vi "ResetDirection.vi"(8 "error in":errorcluster, 11 "class data in":refnum<class "Ball.lvclass">) -> (0 "error out":errorcluster, 3 "class data out":refnum<class "Ball.lvclass">)   [LabVIEW 2010, in "Labricks.lvlib" / "Ball.lvclass"]
uses:
  Ball.lvclass
  properties/InitialDirection/GetInitialDirection.vi
  RenderBase/Sprite_class/properties/Direction/SetDirection.vi
  RenderBase/Sprite_class/Sprite.lvclass
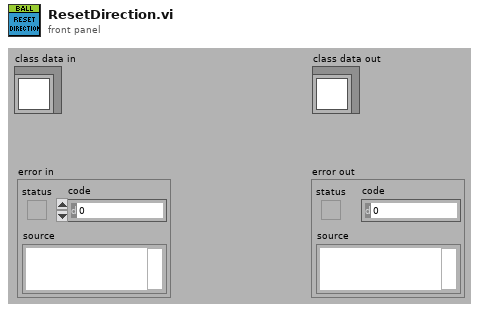
[diagram p1: front panel]
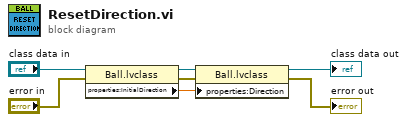
[diagram p0: block diagram]
diagram:
  n1 = property class="Ball.lvclass"(reference="class data in", error in="error in") -> (reference out=w2:refnum<class "Ball.lvclass">, error out=w4:errorcluster, "properties:InitialDirection"=w1:csg)
  n2 = property class="Ball.lvclass"(reference=w2, error in=w4, "properties:Direction"=w1) -> (reference out=→"class data out":refnum<class "Ball.lvclass">, error out=→"error out":errorcluster)
